vi "Register For Listbox Events.vi"(4 "Timeout [ms]":i32=-1, 5 "EventFilter Reference":T1, 6 "Timeout Message (to Self)":refnum<class "Message.lvclass">, 7 "Timeout Message Priority (Normal)":T2=enum."Normal", 8 "error in (no error)":errorcluster, 9 "Registration Types":T3[](array[typedef]), 10 "Listbox Refnum":refnum<vi>, 11 "IEventAggregator In":refnum<class "IEventAggregator.lvclass">) -> (0 "error out":errorcluster, 3 "IEventAggregator Out":refnum<class "IEventAggregator.lvclass">)   [LabVIEW 2017, in "ActorEvents.lvlib" / "IEventAggregator.lvclass"]
uses:
  <vilib>/gpm_packages/@cs/mva-viewable/Source/ActorEvents/IEventAggregator/IEventAggregator.lvclass
  <vilib>/event_ctls.llb/lveventtype.ctl
  <vilib>/ActorFramework/Message/Message.lvclass
  <vilib>/ActorFramework/Message Enqueuer/Message Priority.ctl
  <vilib>/gpm_packages/@cs/mva-viewable/Source/ActorEvents/IEventFilter/EventFilter Reference.ctl
  <vilib>/gpm_packages/@cs/mva-viewable/Source/ActorEvents/IEventFilter/IEventFilter.lvclass
  <vilib>/gpm_packages/@cs/mva-viewable/Source/ActorEvents/IEventHandler/IEventHandler.lvclass/IEventHandler.ctl
  <vilib>/gpm_packages/@cs/mva-viewable/Source/ActorEvents/EventHandler/ListboxEventHandler/ListboxEventHandler.lvclass/ListboxEventHandler.ctl
  <vilib>/gpm_packages/@cs/mva-viewable/Source/ActorEvents/IEventAggregator/IEventAggregator.lvclass/IEventAggregator.ctl
  <vilib>/gpm_packages/@cs/mva-viewable/Source/ActorEvents/IEventHandler/Write Registration Types.vi
  <vilib>/gpm_packages/@cs/mva-viewable/Source/ActorEvents/IEventHandler/Write Timeout Message.vi
  <vilib>/gpm_packages/@cs/mva-viewable/Source/ActorEvents/IEventHandler/Write EventFilter Reference.vi
  <vilib>/gpm_packages/@cs/mva-viewable/Source/ActorEvents/EventHandler/ListboxEventHandler/ListboxEventHandler.lvclass
  C:/Program Files/National Instruments/LabVIEW 2017/vi.lib/gpm_packages/@cs/mva-viewable/Source/ActorEvents/IEventHandler/IEventHandler.lvclass
  <vilib>/Utility/error.llb/Error Cluster From Error Code.vi
  <vilib>/gpm_packages/@cs/mva-viewable/Source/ActorEvents/IEventHandler/IEventHandler.lvclass
  <vilib>/ActorFramework/Message Enqueuer/Message Enqueuer.lvclass
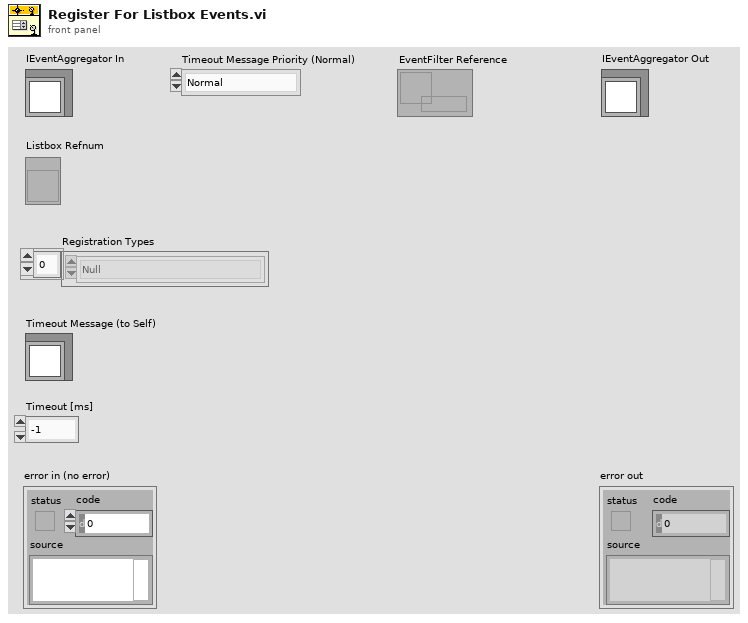
[diagram p1: front panel]
types:
  T1 = typedef "ActorEvents.lvlib/IEventFilter.lvclass/EventFilter Reference.ctl" = refnum<data-value>
  T2 = typedef "Actor Framework.lvlib/Message Enqueuer.lvclass/Message Priority.ctl" = enum16{"Low", "Normal", "High"}
  T3 = typedef "lveventtype.ctl" = enum32{"Null", "Timeout", "Annotation Menu Selection", "Annotation Menu Selection?", "App Instance Close", "App Instance Close?", "Autoscale Range Change", "Bookmark Info Change", "Cell Edit", "Cell Edit?", "Cursor Grab", "Cursor Grab?", "Cursor Menu Selection", "Cursor Menu Selection?", "Cursor Move", "Cursor Release", "Data Change", "Direction Change", "Display State Change", "Drag Ended", "Drag Enter", "Drag Leave", "Drag Over", "Drag Source Update", "Drag Starting", "Drag Starting?", "Drop", "Exec State Change", "Key Down", "Key Down?", "Key Repeat", "Key Repeat?", "Key Up", "Listbox Double Click", "Menu Activation?", "Menu Selection (App)", "Menu Selection? (App)", "Menu Selection (User)", "Mouse Down", "Mouse Down?", "Mouse Enter", "Mouse Leave", "Mouse Move", "Mouse Up", "Mouse Wheel", "NI Security User Change (App)", "Pane Size", "Panel Close", "Panel Close?", "Panel Resize", "Plot Attribute Change", "Scale Range Change", "Shortcut Menu Activation?", "Shortcut Menu Selection (App)", "Shortcut Menu Selection? (App)", "Shortcut Menu Selection (User)", "Tree Double Click", "Tree Drag", "Tree Drag?", "Tree Drop", "Tree Drop?", "Tree Item Close", "Tree Item Close?", "Tree Item Open", "Tree Item Open?", "User Event", "Value Change"}
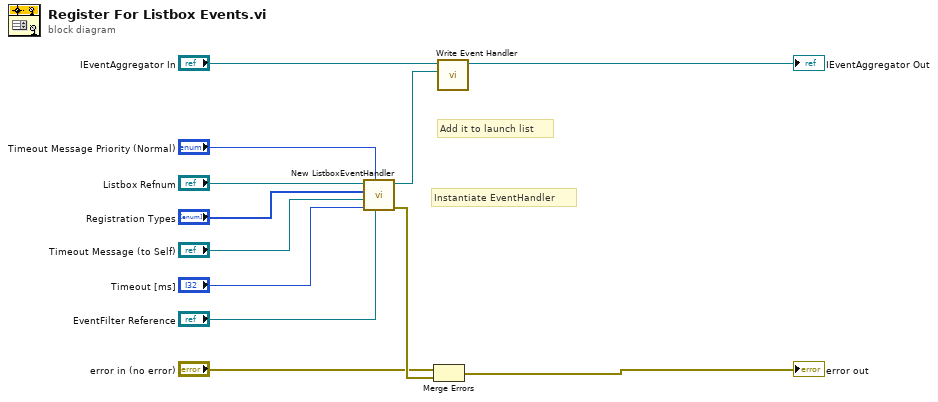
[diagram p0: block diagram]
diagram:
  # "Add it to launch list"
  # "Instantiate EventHandler"
  n1 = call <vilib>:"New ListboxEventHandler.vi"("EventFilter Reference"="EventFilter Reference", "Timeout Message Priority (Normal)"="Timeout Message Priority (Normal)", "Timeout [ms]"="Timeout [ms]", "Timeout Message"="Timeout Message (to Self)", "Registrations"="Registration Types", "Listbox"="Listbox Refnum") -> ("error out"=w12:errorcluster, "ListboxEventHandler"=w1:refnum<class "ListboxEventHandler.lvclass">)  [unwired: 4 in]
  n2 = Merge Errors("error in (no error)", w12) -> (→"error out":errorcluster)
  n3 = call <vilib>:"Write Event Handler.vi"("EventHandler"=w1, "IEventAggregator in"="IEventAggregator In") -> ("IEventAggregator out"=→"IEventAggregator Out":refnum<class "IEventAggregator.lvclass">)  [unwired: 9 in]
